vi "Actor Core.vi"(8 "error in":errorcluster, 11 "HIJ Vision Application in":refnum<class "HIJ Vision Application.lvclass">) -> (0 "error out":errorcluster={"status"=FALSE, "code"=0, "source"="Actor Framework.lvlib:Actor.lvclass:Launch Nested Actor.vi<APPEND>\n\n<b>Complete call chain:</b>\r\n     Actor Framework.lvlib:Actor.lvclass:Launch Nested Actor.vi\r\n     Launch HIJ FileViewer.lvlib:Launch File Viewer.lvclass:Actor Core.vi"}, 3 "Actor out":refnum<class "Actor.lvclass">)   [LabVIEW 2020, in "HIJ Vision Application.lvlib" / "HIJ Vision Application.lvclass"]
doc: "(<B>Filename</B>: Actor Framework.lvlib:Actor.lvclass:Actor Core.vi)\n\nReceives messages to the actor, reacts to them, and initiates any error handling that may shut the actor down.\n\nDescendant classes may override this VI to append parallel tasks for the actor to complete while it handles messages. Overrides use the Call Parent Method node."
uses:
  HIJ Vision Application.lvclass
  HIJ Vision Application.lvclass/HIJ Vision Application.ctl
  Viewable Actor/ViewableActor Messages/Insert Into SubPanel Msg/Insert Into SubPanel Msg.lvclass
  <vilib>/ActorFramework/Actor/Actor.lvclass
  HIJ Vision Application Messages/After Launch Init Msg/After Launch Init Msg.lvclass
  <vilib>/ActorFramework/Message Enqueuer/Message Priority.ctl
  <vilib>/ActorFramework/Message Enqueuer/Message Enqueuer.lvclass
  Analyze/Analyze Actor/Analyze Actor/Analyze Actor.lvclass
  Display Actors/HIJ Vision Display/HIJ Vision Display/HIJ Vision Display.lvclass
  Viewable Actor/ViewableActor/ViewableActor.lvclass
  C:/Users/AlexK/work/LabVIEW Programme/POLARIS-AS-3-Cams/Submodules/Viewable Actor/ViewableActor/ViewableActor.lvclass
  C:/Program Files (x86)/National Instruments/LabVIEW 2020/vi.lib/ActorFramework/Actor/Actor.lvclass
  C:/Users/AlexK/work/LabVIEW Programme/POLARIS-AS-3-Cams/Submodules/HIJ Vision/Application Base Actors/HIJ Vision Application/HIJ Vision Application/HIJ Vision Application.lvclass
  C:/Users/AlexK/work/LabVIEW Programme/POLARIS-AS-3-Cams/Submodules/HIJ Vision/Analyze/Analyze Actor/IAnalysis/IAnalysis.lvclass
  C:/Users/AlexK/work/LabVIEW Programme/POLARIS-AS-3-Cams/Submodules/HIJ Vision/Display Actors/HIJ Vision Display/HIJ Vision Display/HIJ Vision Display.lvclass
  C:/Users/AlexK/work/LabVIEW Programme/POLARIS-AS-3-Cams/Submodules/HIJ Vision/Camera Actors/Camera Actor/ICamera/ICamera.lvclass
  C:/Users/AlexK/work/LabVIEW Programme/POLARIS-AS-3-Cams/Submodules/HIJ Vision/Analyze/Analyze Actor/Analyze Actor/Analyze Actor.lvclass
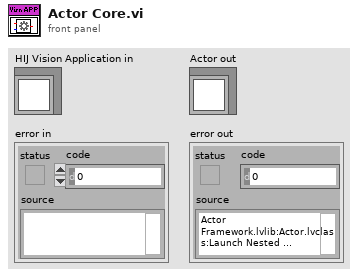
[diagram p1: front panel]
types:
  T1 = typedef "Actor Framework.lvlib/Message Enqueuer.lvclass/Message Priority.ctl" = enum16{"Low", "Normal", "High"}
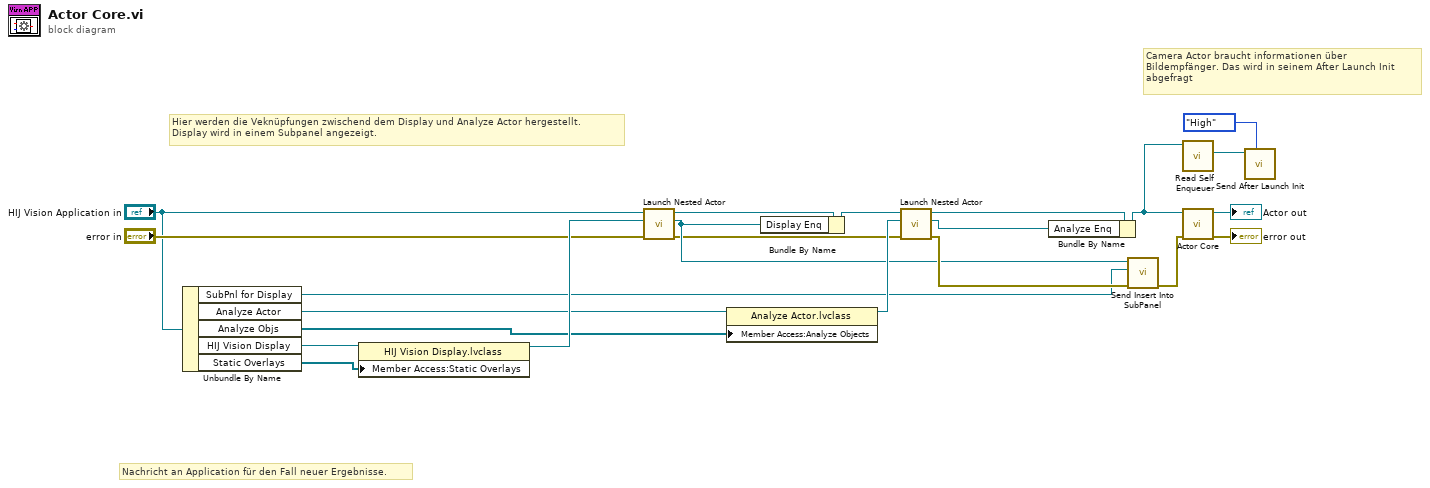
[diagram p0: block diagram]
diagram:
  # "Nachricht an Application für den Fall neuer Ergebnisse."
  # "Camera Actor braucht informationen über\nBildempfänger. Das wird in seinem After Launch Init\nabgefragt"
  # "Hier werden die Veknüpfungen zwischend dem Display und Analyze Actor hergestellt.\nDisplay wird in einem Subpanel angezeigt."
  n1 = Unbundle By Name("HIJ Vision Application in") -> ("SubPnl for Display"=w1:refnum<vi>, "Analyze Actor"=w3:refnum<class "Analyze Actor.lvclass">, "Analyze Objs"=w4:refnum<class "Analyze BaseClass.lvclass">[], "HIJ Vision Display"=w7:refnum<class "HIJ Vision Display.lvclass">, "Static Overlays"=w6:refnum<class "Static Overlay.lvclass">[])
  n2 = property class="HIJ Vision Display.lvclass"(reference=w7, "Member Access:Static Overlays"=w6) -> (reference out=w22:refnum<class "HIJ Vision Display.lvclass">)  [unwired: 1 in, 1 out]
  n3 = call <vilib>:"Launch Nested Actor.vi"("error in (no error)"="error in", "Nested Actor"=w22, "Caller Actor in"="HIJ Vision Application in") -> ("error out"=w2:errorcluster, "Nested Actor's Enqueuer"=w5:refnum<class "Message Enqueuer.lvclass">, "Caller Actor out"=w18:refnum<class "HIJ Vision Application.lvclass">)  [unwired: 6 in]
  n4 = property class="Analyze Actor.lvclass"(reference=w3, "Member Access:Analyze Objects"=w4) -> (reference out=w17:refnum<class "Analyze Actor.lvclass">)  [unwired: 1 in, 1 out]
  n5 = Bundle By Name(cluster=w18, "Display Enq"=w5) -> (w10:refnum<class "HIJ Vision Application.lvclass">)
  n6 = call <vilib>:"Launch Nested Actor.vi"("error in (no error)"=w2, "Nested Actor"=w17, "Caller Actor in"=w10) -> ("error out"=w16:errorcluster, "Nested Actor's Enqueuer"=w8:refnum<class "Message Enqueuer.lvclass">, "Caller Actor out"=w13:refnum<class "HIJ Vision Application.lvclass">)  [unwired: 6 in]
  n7 = Bundle By Name(cluster=w13, "Analyze Enq"=w8) -> (w9:refnum<class "HIJ Vision Application.lvclass">)
  n8 = call "Send Insert Into SubPanel.vi"("error in (no error)"=w16, "SubPanel Ref"=w1, "Message Enqueuer"=w5) -> ("error out"=w15:errorcluster)  [unwired: 7 in, 1 out]
  n9 = call <vilib>:"Read Self Enqueuer.vi"("Actor"=w9) -> ("Self Enqueuer"=w12:refnum<class "Message Enqueuer.lvclass">)  [unwired: 10 in]
  n10 = call-parent "Actor Core.vi"("error in"=w15, "Actor in"=w9) -> ("error out"=→"error out":errorcluster, "Actor out"=→"Actor out":refnum<class "Actor.lvclass">)  [unwired: 8 in]
  n11 = call "Send After Launch Init.vi"("Message Priority (Normal)"=Message_Priority."High", "Message Enqueuer"=w12) -> ()  [unwired: 8 in, 2 out]
